vi "Report Error.vi"(8 "error in":errorcluster, 11 "Status":refnum<vi>) -> (0 "error out":errorcluster)   [LabVIEW 2014, in "Raspberry Pi Compatible Compiler for LabVIEW.lvlib"]
uses:
  Raspberry Pi Compatible Compiler for LabVIEW.lvlib
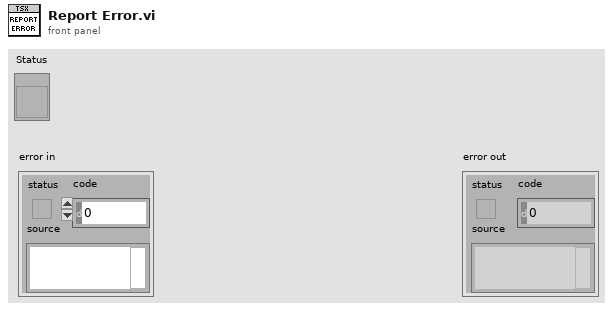
[diagram p1: front panel]
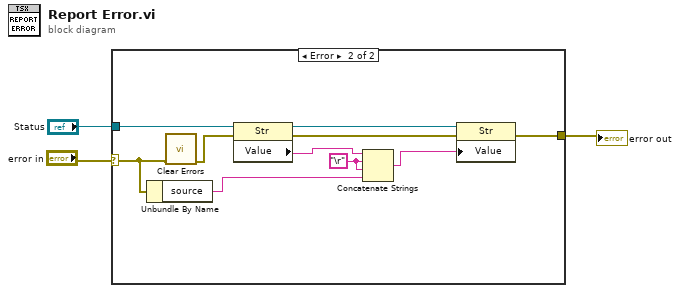
[diagram p0: block diagram]
diagram:
  n1 = case shown="Error" "error in" {
    selector: "error in" -> [w4 w9]
    tunnel: "Status" -> [_ w13]
    tunnel: [w4 w14] -> w1
    frame No Error {
    }
    frame Error {
      w6 = "\r"
      n2 = Unbundle By Name(w9) -> ("source"=w5:string)
      n3 = call <vilib>:"Clear Errors.vi"("error in (no error)"=w9) -> ("error out"=w10:errorcluster)  [unwired: 5 in, 1 out]
      n4 = property class="Str"(reference=w13, error in=w10) -> (reference out=w12:refnum<vi>, error out=w8:errorcluster, "Value"=w7:string)
      n5 = Concatenate Strings(w7, w6, w6, w5) -> (w11:string)
      n6 = property class="Str"(reference=w12, error in=w8, "Value"=w11) -> (error out=w14:errorcluster)  [unwired: 1 out]
    }
  }
  "error out" <- w1
